vi "PathPlanner_EventMarker_FromJSON.vi"(11 "JSON String":string) -> (0 "Exists":bool, 3 "EventMarkers":T2[](array[typedef]))   [LabVIEW 2019, in "PathPlanner24.lvlib"]
doc: "Create a list of event markers from json string\n\nInputs:\n - JSONString - string - String potentially containing an event marker\n\nOutputs:\n - EventMarkers - array of cluster - The event markers defined by the given json object\n - Exists - boolean- TRUE if any event markers were found in the JSON string.\n\nNotes:\n--------\nCurrently the only type of commands that can be issued are Boolean commands. The value is forced to TRUE when the command is issued.\n\nThe following table lists the actions performed for different types of commands:\n - Unknown - nothing - not supported.\n - Wait - nothing - not supported\n - Named - Issue boolean command with TRUE value using the \"name\" as the command name.\n - Path - nothing - not supported\n - Sequential, Parallel, Race, Deadline - Issue boolean command with TRUE value for each of the commands contained in the \"commands\" array. The value for \"name\" is used as the command name."
uses:
  PathPlanner24.lvlib
  TypeDef/PathPlannerEventMarker.ctl
  TypeDef/PathPlannerCommandUtil.ctl
  ENum/PathPlanner_CommandUtil_Type_ENUM.ctl
panel:
  in  "eventMarkers":T1(array[cluster])
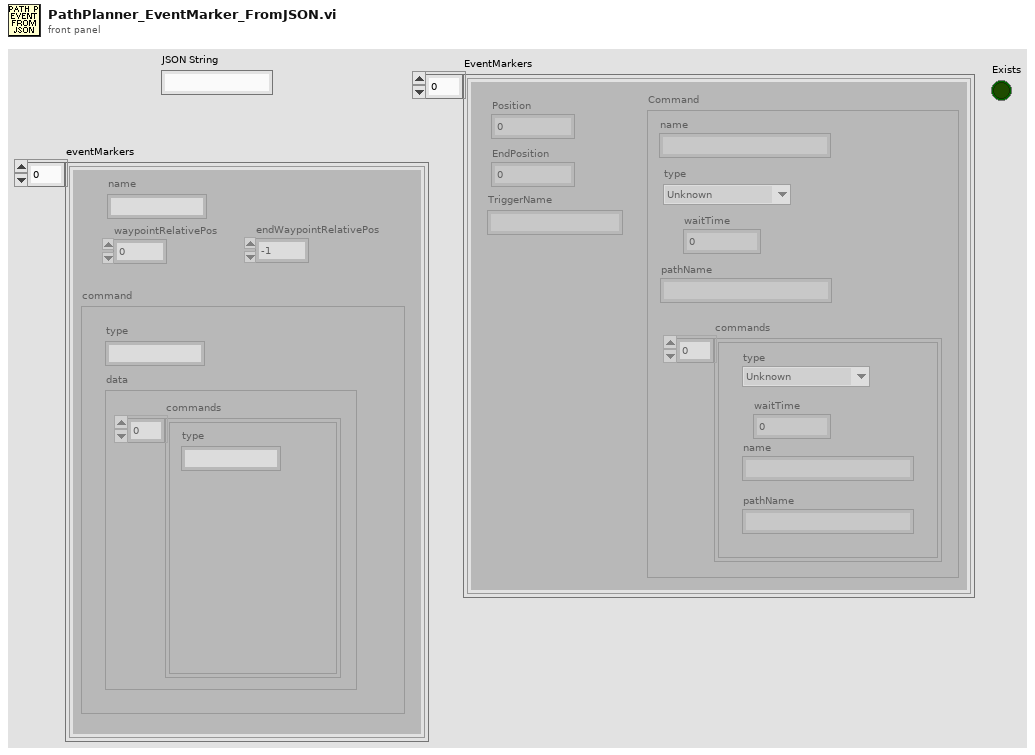
[diagram p1: front panel]
types:
  T1 = cluster{"name":string, "waypointRelativePos":dbl, "command":cluster{"type":string, "data":cluster{"commands":cluster{"type":string}[]}}, "endWaypointRelativePos":dbl}[]
  T2 = typedef "PathPlanner24.lvlib/PathPlannerEventMarker.ctl" = cluster{"Position":dbl, "Command":T3, "TriggerName":string, "EndPosition":dbl}
  T3 = typedef "PathPlanner24.lvlib/PathPlannerCommandUtil.ctl" = cluster{"waitTime":dbl, "name":string, "pathName":string, "commands":cluster{"type":T4, "waitTime":dbl, "name":string, "pathName":string}[], "type":T4}
  T4 = typedef "PathPlanner24.lvlib/PathPlanner_CommandUtil_Type_ENUM.ctl" = enum16{"Unknown", "Wait", "Named", "Path", "Sequential", "Parallel", "Race", "Deadline"}
  T5 = cluster{"type":T4, "waitTime":dbl, "name":string, "pathName":string}
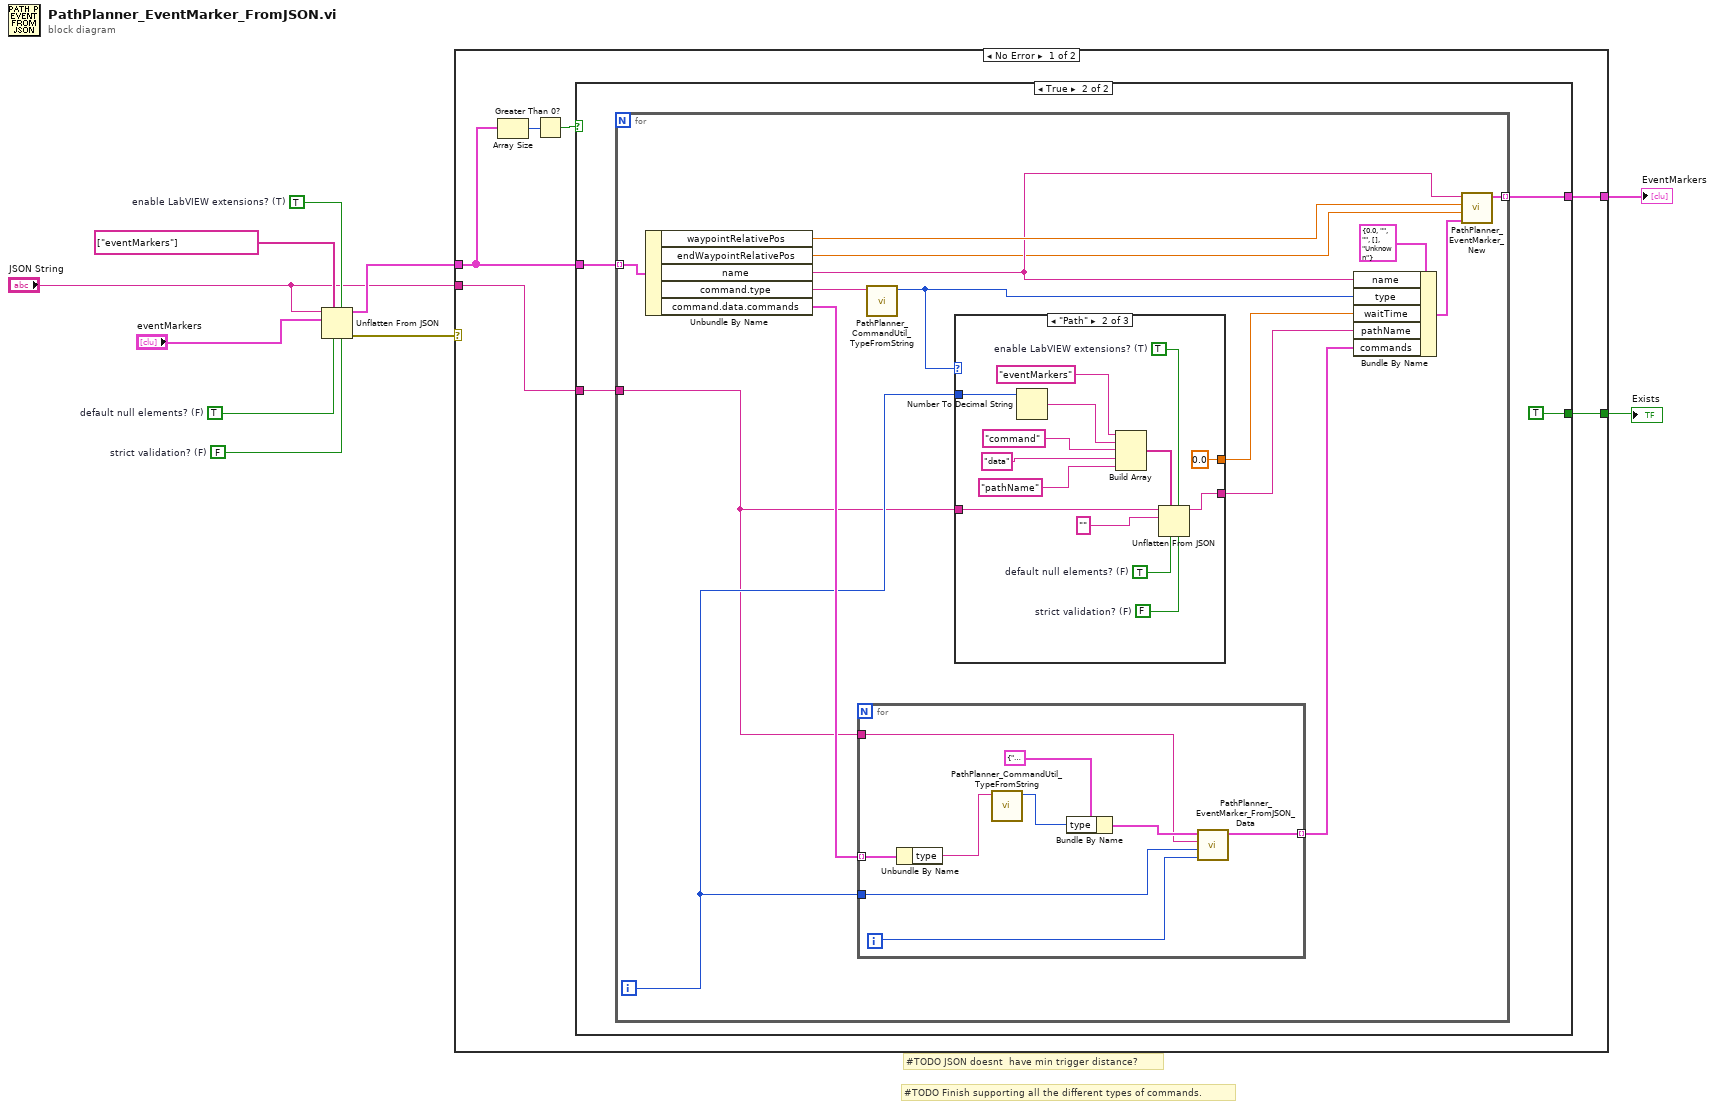
[diagram p0: block diagram]
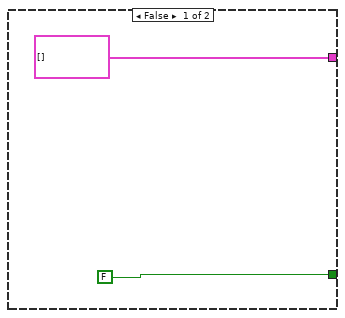
[diagram p2: hidden frame]
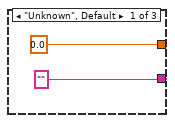
[diagram p3: hidden frame]
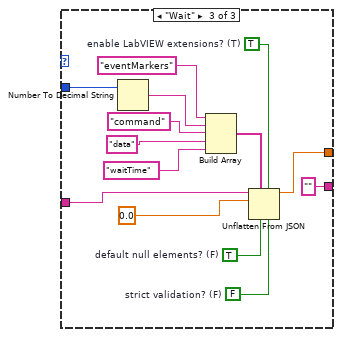
[diagram p4: hidden frame]
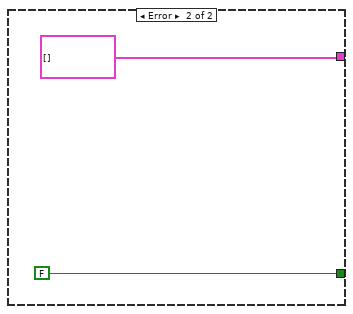
[diagram p5: hidden frame]
diagram:
  w7 = FALSE  # strict validation? (F)
  w8 = TRUE  # default null elements? (F)
  w9 = TRUE  # enable LabVIEW extensions? (T)
  # "#TODO Finish supporting all the different types of commands."
  # "#TODO JSON doesnt  have min trigger distance?"
  n1 = Unflatten From JSON(path=string[] ["eventMarkers"] ("path 2"), enable LabVIEW extensions? (T)=w9, JSON string="JSON String", type and defaults="eventMarkers", default null elements? (F)=w8, strict validation? (F)=w7) -> (value=w5:T1, error out=w6:errorcluster)  [unwired: 1 in]
  n2 = case shown="No Error" w6 {
    tunnel: w5 -> [w14 _]
    tunnel: [w12 FALSE] -> w3
    tunnel: [w13 T2[] []] -> w2
    tunnel: "JSON String" -> [w11 _]
    frame No Error {
      n3 = Array Size(array=w14) -> (size(s)=w16:i32)
      n4 = Greater Than 0?(x=w16) -> (x > 0?=w15:bool)
      n5 = case shown="True" w15 {
        tunnel: w14 -> [_ w22]
        tunnel: [T2[] [] w21] -> w13
        tunnel: [FALSE TRUE] -> w12
        tunnel: w11 -> [_ w19]
        frame False {
        }
        frame True {
          n6 = for {
            tunnel: w22 -> [w37] mode=indexing
            tunnel: [w34] -> w21 mode=indexing
            tunnel: w19 -> [w25]
            i -> [w26]
            n7 = Unbundle By Name(w37) -> ("waypointRelativePos"=w30:dbl, "endWaypointRelativePos"=w28:dbl, "name"=w29:string, "command.type"=w33:string, "command.data.commands"=w35:cluster{"type":string}[])
            n8 = for {
              tunnel: w35 -> [w76] mode=indexing
              tunnel: [w71] -> w32 mode=indexing
              tunnel: w25 -> [w70]
              tunnel: w26 -> [w69]
              i -> [w68]
              n9 = Unbundle By Name(w76) -> ("type"=w74:string)
              n10 = call "PathPlanner_CommandUtil_TypeFromString.vi"("Type string"=w74) -> ("Type"=w75:T4)  [unwired: 10 in]
              n11 = Bundle By Name(cluster=T5 {"type"=enum."Unknown", "waitTime"=0.0, "name"="", "pathName"=""} ("Command"), "type"=w75) -> (w72:T5)
              n12 = call "PathPlanner_EventMarker_FromJSON_Data.vi"("Cmd Index"=w68, "Index"=w69, "JSON String"=w70, "In Command Data"=w72) -> ("out Command Data"=w71:T5)  [unwired: 6 in, 1 out]
            }
            n13 = call "PathPlanner_CommandUtil_TypeFromString.vi"("Type string"=w33) -> ("Type"=w27:T4)  [unwired: 10 in]
            n14 = case shown="\"Path\"" w27 {
              tunnel: w25 -> [_ w49 w60]
              tunnel: ["" w44 ""] -> w23
              tunnel: [0.0 0.0 w58] -> w24
              tunnel: w26 -> [_ w41 w56]
              frame "Unknown", Default {
              }
              frame "Path" {
                w51 = FALSE  # strict validation? (F)
                w52 = TRUE  # default null elements? (F)
                w53 = TRUE  # enable LabVIEW extensions? (T)
                n15 = Number To Decimal String(number=w41) -> (decimal integer string=w40:string)  [unwired: 1 in]
                n16 = Build Array("eventMarkers", w40, "command", "data", "pathName") -> (w48:string[])
                n17 = Unflatten From JSON(path=w48, enable LabVIEW extensions? (T)=w53, JSON string=w49, type and defaults="", default null elements? (F)=w52, strict validation? (F)=w51) -> (value=w44:string)  [unwired: 1 in, 1 out]
              }
              frame "Wait" {
                w65 = FALSE  # strict validation? (F)
                w66 = TRUE  # default null elements? (F)
                w67 = TRUE  # enable LabVIEW extensions? (T)
                n18 = Number To Decimal String(number=w56) -> (decimal integer string=w55:string)  [unwired: 1 in]
                n19 = Build Array("eventMarkers", w55, "command", "data", "waitTime") -> (w64:string[])
                n20 = Unflatten From JSON(path=w64, enable LabVIEW extensions? (T)=w67, JSON string=w60, type and defaults=0.0, default null elements? (F)=w66, strict validation? (F)=w65) -> (value=w58:dbl)  [unwired: 1 in, 1 out]
              }
            }
            n21 = Bundle By Name(cluster=T3 {"waitTime"=0.0, "name"="", "pathName"="", "commands"=[], "type"=enum."Unknown"} ("Command"), "name"=w29, "type"=w27, "waitTime"=w24, "pathName"=w23, "commands"=w32) -> (w31:T3)
            n22 = call "PathPlanner_EventMarker_New.vi"("Command"=w31, "EndPosition"=w28, "Position"=w30, "TriggerName"=w29) -> ("EventMarker"=w34:T2)  [unwired: 7 in]
          }
        }
      }
    }
    frame Error {
    }
  }
  "EventMarkers" <- w2
  "Exists" <- w3
